vi "KH_config.vi"(8 "Error In":errorcluster, 9 "Function":enum16{"write", "read"}(ring), 10 "Gains":dbl[](array[numeric]), 11 "Channel Setting":T1) -> (0 "Error Out":errorcluster, 2 "Gains out":dbl[](array[numeric]), 3 "Channel Setting":T1)   [LabVIEW 2019, in "Instrument.KH7008.lvclass"]
uses:
  Instrument.KH7008.lvclass
  typedefs/SetAll-Array.ctl
  typedefs/SetAll-Cluster.ctl
  typedefs/Channel-Enum.ctl
  typedefs/Gain-Enum.ctl
  typedefs/Filter-Enum.ctl
  typedefs/Shunt-Enum.ctl
  typedefs/Coupling-Enum.ctl
  typedefs/Input Configuration-Enum.ctl
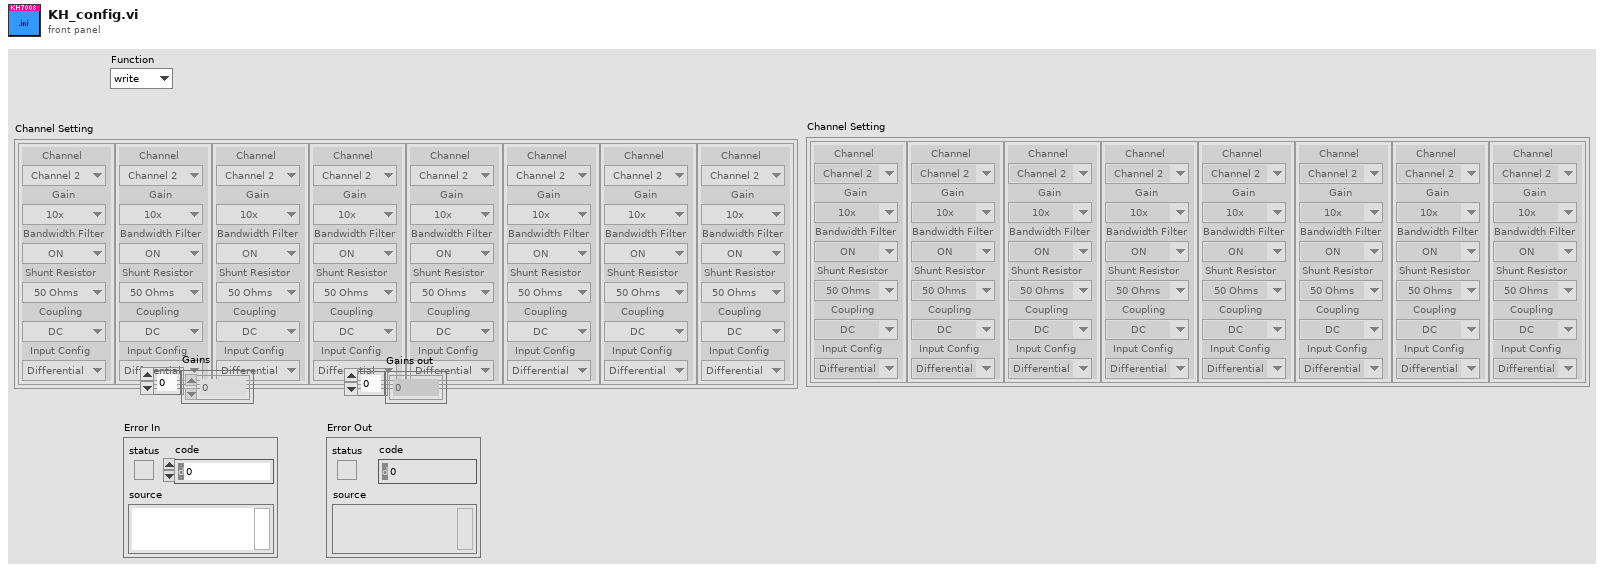
[diagram p1: front panel]
types:
  T1 = typedef "Instrument.KH7008.lvclass/SetAll-Array.ctl" = T2[]
  T2 = typedef "Instrument.KH7008.lvclass/SetAll-Cluster.ctl" = cluster{"Channel":T3, "Gain":T4, "Bandwidth Filter":T5, "Shunt Resistor":T6, "Coupling":T7, "Input Config":T8}
  T3 = typedef "Instrument.KH7008.lvclass/Channel-Enum.ctl" = enum16{"Channel 1", "Channel 2", "Channel 3", "Channel 4", "Channel 5", "Channel 6", "Channel 7", "Channel 8"}
  T4 = typedef "Instrument.KH7008.lvclass/Gain-Enum.ctl" = enum16{"1x", "10x", "100x", "1000x"}
  T5 = typedef "Instrument.KH7008.lvclass/Filter-Enum.ctl" = enum16{"OFF", "ON"}
  T6 = typedef "Instrument.KH7008.lvclass/Shunt-Enum.ctl" = enum16{"Open", "50 Ohms", "500 Ohms", "5k Ohms", "50k Ohms", "10M Ohm"}
  T7 = typedef "Instrument.KH7008.lvclass/Coupling-Enum.ctl" = enum16{"AC", "DC"}
  T8 = typedef "Instrument.KH7008.lvclass/Input Configuration-Enum.ctl" = enum16{"Ground", "SE+ (-gnd)", "SE- (+gnd)", "Differential"}
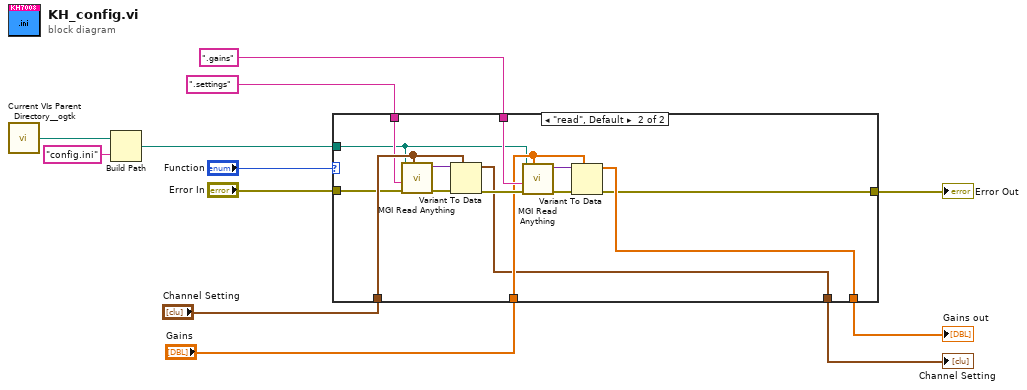
[diagram p0: block diagram]
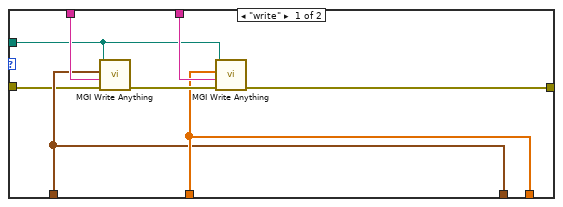
[diagram p2: hidden frame]
diagram:
  n1 = call <userlib>:"Current VIs Parent Directory__ogtk.vi"() -> ("Parent Directory (+ Relative)"=w12:path)  [unwired: 5 in]
  n2 = Build Path(base path=w12, name or relative path="config.ini") -> (appended path=w10:path)
  n3 = case shown="\"read\", Default" "Function" {
    tunnel: ".settings" ("Section Name (Name of \"Anything\")") -> [w20 w29]
    tunnel: "Gains" -> [w16 w27]
    tunnel: ".gains" ("Section Name (Name of \"Anything\")") -> [w18 w28]
    tunnel: "Channel Setting" -> [w15 w32]
    tunnel: w10 -> [w17 w25]
    tunnel: [w14 w21] -> w9
    tunnel: "Error In" -> [w13 w26]
    tunnel: [w15 w24] -> w3
    tunnel: [w16 w23] -> w2
    frame "write" {
      n4 = call <userlib>:"MGI Write Anything.vi"("Error In"=w13, "Section Name (Name of \"Anything\")"=w20, "Anything"=w15, "Path (dialog)"=w17) -> ("Error Out"=w19:errorcluster)  [unwired: 5 in, 2 out]
      n5 = call <userlib>:"MGI Write Anything.vi"("Error In"=w19, "Section Name (Name of \"Anything\")"=w18, "Anything"=w16, "Path (dialog)"=w17) -> ("Error Out"=w14:errorcluster)  [unwired: 5 in, 2 out]
    }
    frame "read", Default {
      n6 = call <userlib>:"MGI Read Anything.vi"("Type of Anything"=w32, "Error In"=w26, "Section Name (Name of \"Type of Anything\")"=w29, "Path (dialog)"=w25) -> ("Error Out"=w34:errorcluster, "Anything"=w33:variant)  [unwired: 4 in, 2 out]
      n7 = Variant To Data(error in=w34, type=w32, Variant=w33) -> (data=w24:T1, error out=w30:errorcluster)
      n8 = call <userlib>:"MGI Read Anything.vi"("Type of Anything"=w27, "Error In"=w30, "Section Name (Name of \"Type of Anything\")"=w28, "Path (dialog)"=w25) -> ("Error Out"=w31:errorcluster, "Anything"=w22:variant)  [unwired: 4 in, 2 out]
      n9 = Variant To Data(error in=w31, type=w27, Variant=w22) -> (data=w23:dbl[], error out=w21:errorcluster)
    }
  }
  "Error Out" <- w9
  "Channel Setting" <- w3
  "Gains out" <- w2
